vi "Signal Breakout.vi"(0 "Pumps Enabled":bool[](array[boolean]), 5 "Tank Data":dbl[](array[numeric]), 7 "Intitial Times":dbl[](array[numeric])) -> (4 "Pump Data":T2={"Voltages"=[0.015201568603515625, 0.00335693359375, 0.003021240234375, 0.12260055541992188, 0.06085968017578125, 0.052234649658203125], "PumpCurrent"=[0.015201568603515625, 0.00335693359375, 0.003021240234375, 0.12260055541992188, 0.06085968017578125, 0.052234649658203125], "Speed"=[0.0, 0.0, 0.0, 0.0, 0.0, 0.0], "ControllerCurrent"=[0.015201568603515625, 0.00335693359375, 0.003021240234375, 0.12260055541992188, 0.06085968017578125, 0.052234649658203125], "Pressure"=[0.015201568603515625, 0.00335693359375, 0.003021240234375, 0.12260055541992188, 0.06085968017578125, 0.052234649658203125], "Flow"=[0.0, 0.0, 0.0, 0.125, 0.0625, 0.0625], "Elapsed Time (Display)"=[7.1, 7.1, 7.1, 458133.45, 458138.85000000003, 458126.75], "Avg Pressure"=0.0, "Avg Speed"=0.0, "Elapsed Time"=[4074.9003000000002, 4074.9003000000002, 4074.9003000000002, 4074.9003000000002, 4074.9003000000002, 4074.9003000000002]} {"Elapsed Time" format="%<%H:%M:%S>t"; "Elapsed Time (Display)" format="%<%H:%M:%S>t"; "Speed" format="%#_4f"; "ControllerCurrent" format="%#.1g"; "Pressure" format="%#.0f"; "Flow" format="%#.0f"; "PumpCurrent" format="%#.1g"; "Voltages" format="%#.0f"}, 6 "Tank Data":T1 {"PS Actual (V):" format="%.2f"; "Temp1" format="%#_2g"; "Temp2" format="%#_2g"})   [LabVIEW 2019]
uses:
  Controls/Pump Data.ctl
  Controls/Tank Data.ctl
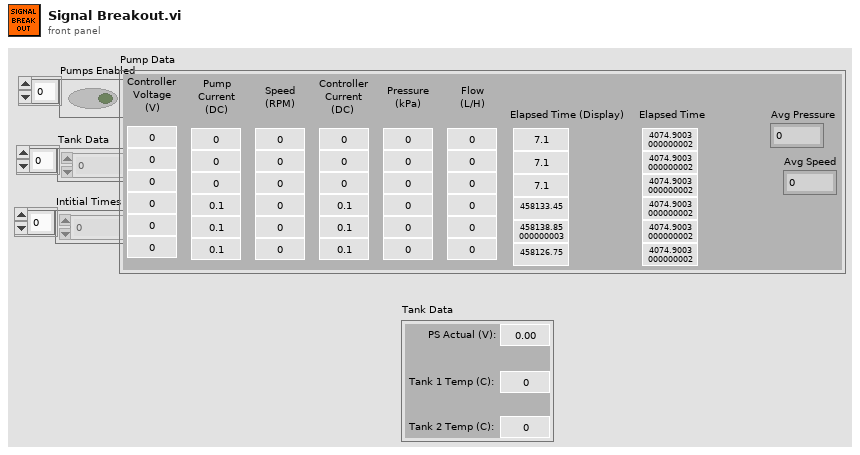
[diagram p1: front panel]
types:
  T1 = typedef "Tank Data.ctl" = cluster{"PS Actual (V):":dbl, "Temp1":dbl, "Temp2":dbl}
  T2 = typedef "Pump Data.ctl" = cluster{"Voltages":dbl[], "PumpCurrent":dbl[], "Speed":dbl[], "ControllerCurrent":dbl[], "Pressure":dbl[], "Flow":dbl[], "Elapsed Time (Display)":dbl[], "Avg Pressure":dbl, "Avg Speed":dbl, "Elapsed Time":dbl[]}
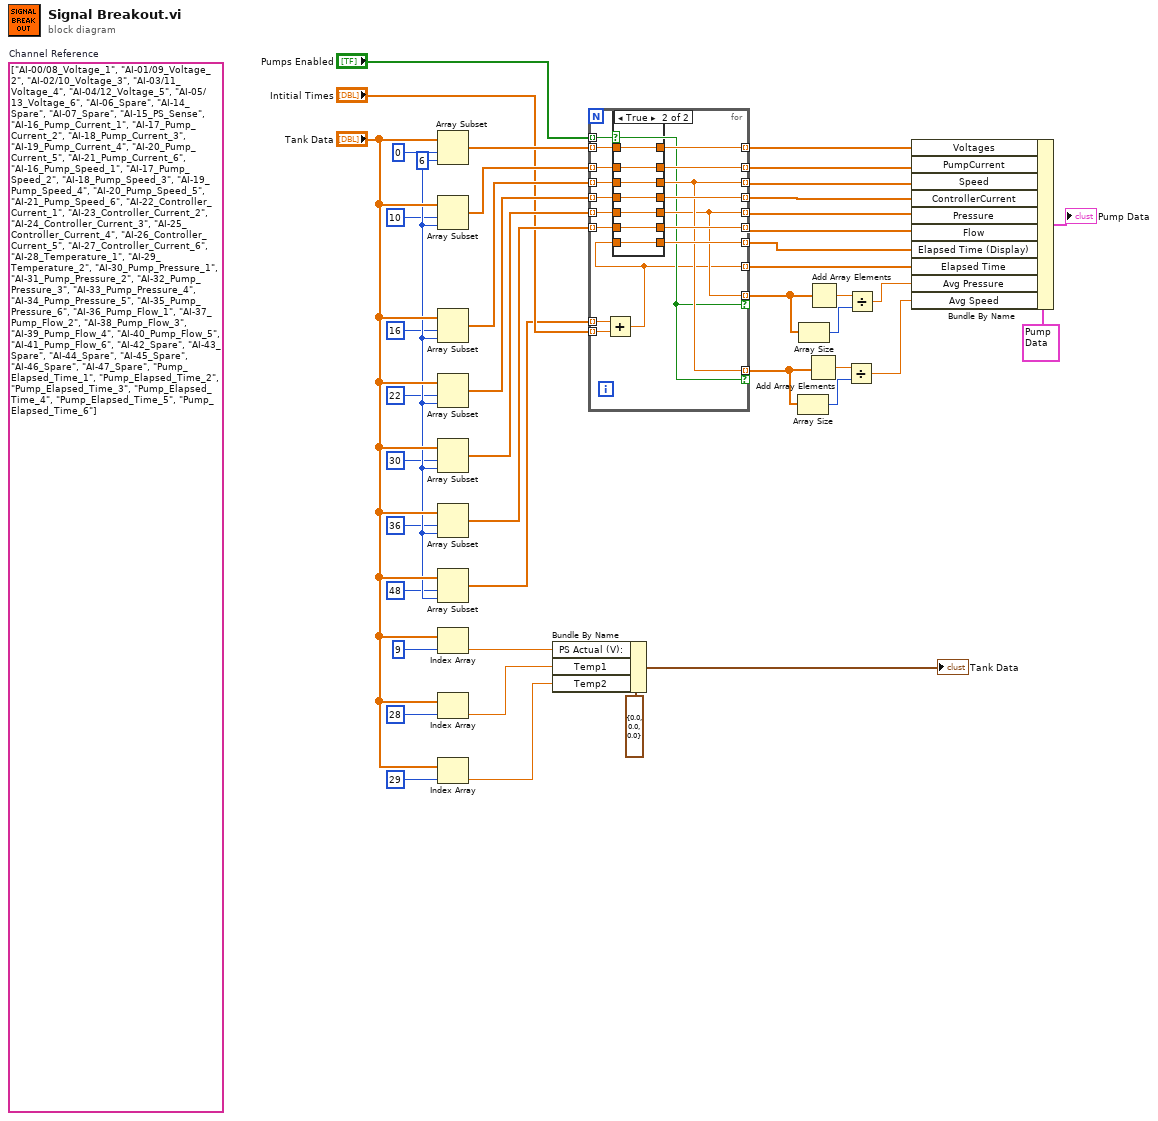
[diagram p0: block diagram]
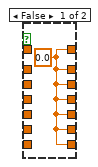
[diagram p2: hidden frame]
diagram:
  w42 = 6 ("length")
  (unwired) string[] ["AI-00/08_Voltage_1", "AI-01/09_Voltage_2", "AI-02/10_Voltage_3", "AI-03/11_Voltage_4", "AI-04/12_Voltage_5", "AI-05/13_Voltage_6", "AI-06_Spare", "AI-14_Spare", "AI-07_Spare", "AI-15_PS_Sense", "AI-16_Pump_Current_1", "AI-17_Pump_Current_2", "AI-18_Pump_Current_3", "AI-19_Pump_Current_4", "AI-20_Pump_Current_5", "AI-21_Pump_Current_6", "AI-16_Pump_Speed_1", "AI-17_Pump_Speed_2", "AI-18_Pump_Speed_3", "AI-19_Pump_Speed_4", "AI-20_Pump_Speed_5", "AI-21_Pump_Speed_6", "AI-22_Controller_Current_1", "AI-23_Controller_Current_2", "AI-24_Controller_Current_3", "AI-25_Controller_Current_4", "AI-26_Controller_Current_5", "AI-27_Controller_Current_6", "AI-28_Temperature_1", "AI-29_Temperature_2", "AI-30_Pump_Pressure_1", "AI-31_Pump_Pressure_2", "AI-32_Pump_Pressure_3", "AI-33_Pump_Pressure_4", "AI-34_Pump_Pressure_5", "AI-35_Pump_Pressure_6", "AI-36_Pump_Flow_1", "AI-37_Pump_Flow_2", "AI-38_Pump_Flow_3", "AI-39_Pump_Flow_4", "AI-40_Pump_Flow_5", "AI-41_Pump_Flow_6", "AI-42_Spare", "AI-43_Spare", "AI-44_Spare", "AI-45_Spare", "AI-46_Spare", "AI-47_Spare", "Pump_Elapsed_Time_1", "Pump_Elapsed_Time_2", "Pump_Elapsed_Time_3", "Pump_Elapsed_Time_4", "Pump_Elapsed_Time_5", "Pump_Elapsed_Time_6"]  # Channel Reference
  n1 = Array Subset(array="Tank Data", index=0, length=w42) -> (w32:dbl[])
  n2 = Array Subset(array="Tank Data", index=10, length=w42) -> (w31:dbl[])
  n3 = Array Subset(array="Tank Data", index=16, length=w42) -> (w30:dbl[])
  n4 = Array Subset(array="Tank Data", index=22, length=w42) -> (w29:dbl[])
  n5 = Array Subset(array="Tank Data", index=30, length=w42) -> (w28:dbl[])
  n6 = Array Subset(array="Tank Data", index=36, length=w42) -> (w27:dbl[])
  n7 = Array Subset(array="Tank Data", index=48, length=w42) -> (w16:dbl[])
  n8 = Index Array(array="Tank Data", index=9) -> (element=w14:dbl)
  n9 = Index Array(array="Tank Data", index=28) -> (element=w13:dbl)
  n10 = Index Array(array="Tank Data", index=29) -> (element=w12:dbl)
  n11 = Bundle By Name(cluster=T1 {"PS Actual (V):"=0.0, "Temp1"=0.0, "Temp2"=0.0} ("Tank Data"), "PS Actual (V):"=w14, "Temp1"=w13, "Temp2"=w12) -> (→"Tank Data":T1)
  n12 = for {
    tunnel: w32 -> [w61] mode=indexing
    tunnel: [w60] -> w23 mode=indexing
    tunnel: w31 -> [w59] mode=indexing
    tunnel: w30 -> [w58] mode=indexing
    tunnel: w29 -> [w57] mode=indexing
    tunnel: w28 -> [w56] mode=indexing
    tunnel: w27 -> [w55] mode=indexing
    tunnel: w16 -> [w51] mode=indexing
    tunnel: [w54] -> w22 mode=indexing
    tunnel: [w48] -> w21 mode=indexing
    tunnel: [w53] -> w20 mode=indexing
    tunnel: [w47] -> w19 mode=indexing
    tunnel: [w52] -> w18 mode=indexing
    tunnel: "Pumps Enabled" -> [w46] mode=indexing
    tunnel: "Intitial Times" -> [w50] mode=indexing
    tunnel: [w49] -> w17 mode=indexing
    tunnel: [w48] -> w3 mode=indexing if=w46
    tunnel: [w47] -> w4 mode=indexing if=w46
    tunnel: [w45] -> w1 mode=indexing
    n13 = Add(x=w51, y=w50) -> (x+y=w45:dbl)
    n14 = case shown="True" w46 {
      tunnel: w61 -> [_ w69]
      tunnel: [w62 w69] -> w60
      tunnel: w59 -> [_ w68]
      tunnel: w58 -> [_ w67]
      tunnel: w57 -> [_ w66]
      tunnel: w56 -> [_ w65]
      tunnel: w55 -> [_ w64]
      tunnel: [w62 w68] -> w54
      tunnel: [w62 w67] -> w48
      tunnel: [w62 w66] -> w53
      tunnel: [w62 w65] -> w47
      tunnel: [w62 w64] -> w52
      tunnel: [w62 w63] -> w49
      tunnel: w45 -> [_ w63]
      frame False {
        w62 = 0.0
      }
      frame True {
      }
    }
  }
  n15 = Array Size(array=w3) -> (size(s)=w6:i32)
  n16 = Array Size(array=w4) -> (size(s)=w8:i32)
  n17 = Add Array Elements(numeric array=w3) -> (sum=w5:dbl)
  n18 = Add Array Elements(numeric array=w4) -> (sum=w9:dbl)
  n19 = Divide(x=w5, y=w6) -> (x/y=w2:dbl)
  n20 = Divide(x=w9, y=w8) -> (x/y=w7:dbl)
  n21 = Bundle By Name(cluster=T2 {"Voltages"=[0.0, 0.05908203125, 0.06982421875, 0.05908203125, 0.06982421875, 0.0859375], "PumpCurrent"=[0.0015967955457961394, 0.0015950073791676203, 0.0015981739242389562, 0.0015920643549248493, 0.001590499709124895, 0.0015808510600251774], "Speed"=[0.0, 0.0, 0.0, 0.0, 0.0, 0.0], "ControllerCurrent"=[-20.688123176070036, -20.81007435196841, -20.6654170362211, -20.809705989642936, -20.754042150663764, -20.945938358319978], "Pressure"=[172.64492233694307, 172.85003218327398, 196.83234134789615, 194.272392502873, 196.0868331665868, 197.0256255267641], "Flow"=[114.82946701905468, 115.15906524483574, 115.40397142867363, 115.72441088850422, 113.53169391236554, 111.97984467984668], "Elapsed Time (Display)"=[4074.9003000000002, 4074.9003000000002, 4074.9003000000002, 4074.9003000000002, 4074.9003000000002, 4074.9003000000002], "Avg Pressure"=0.0, "Avg Speed"=0.0, "Elapsed Time"=[]} ("Pump Data"), "Voltages"=w23, "PumpCurrent"=w22, "Speed"=w21, "ControllerCurrent"=w20, "Pressure"=w19, "Flow"=w18, "Elapsed Time (Display)"=w17, "Elapsed Time"=w1, "Avg Pressure"=w7, "Avg Speed"=w2) -> (→"Pump Data":T2)
